vi "PC_COUNT_ALL_SS_1.vi"(0 "Refnum in":T1, 1 "data in":string[][](array[string]), 3 "Array 3":string[](array[string]), 5 "To Date":string, 9 "From Date":string, 11 "error in (no error)":errorcluster, 12 "Station":string[](array[string])=["1", "2", "3", "4", "5", "6"], 14 "Shift":string[](array[string])=["1", "2", "3", "4", "5", "6"]) -> (4 "Refnum out":T1, 6 "data out":string[][](array[string]), 8 "DATE":string[](array[string]), 10 "COUNT":string[](array[string]), 15 "error out":errorcluster)   [LabVIEW 2017]
uses:
  <vilib>/addons/database/Connection.llb/Conn ObjectReference.ctl
  <vilib>/addons/database/NI_Database_API.lvlib
panel:
  in  "STATION":i32[](array[numeric])
  in  "SHIFT":i32[](array[numeric])
  in  "From Date":timestamp
  in  "To Date":timestamp
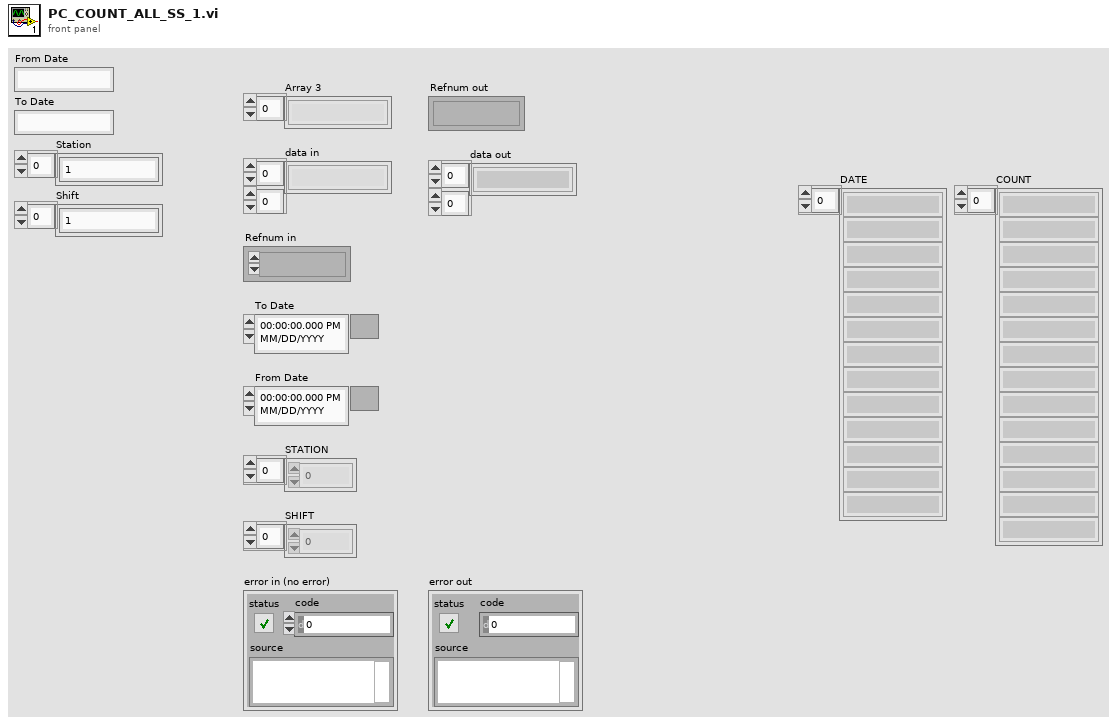
[diagram p1: front panel]
types:
  T1 = typedef "NI_Database_API.lvlib/Conn ObjectReference.ctl" = refnum<k1>
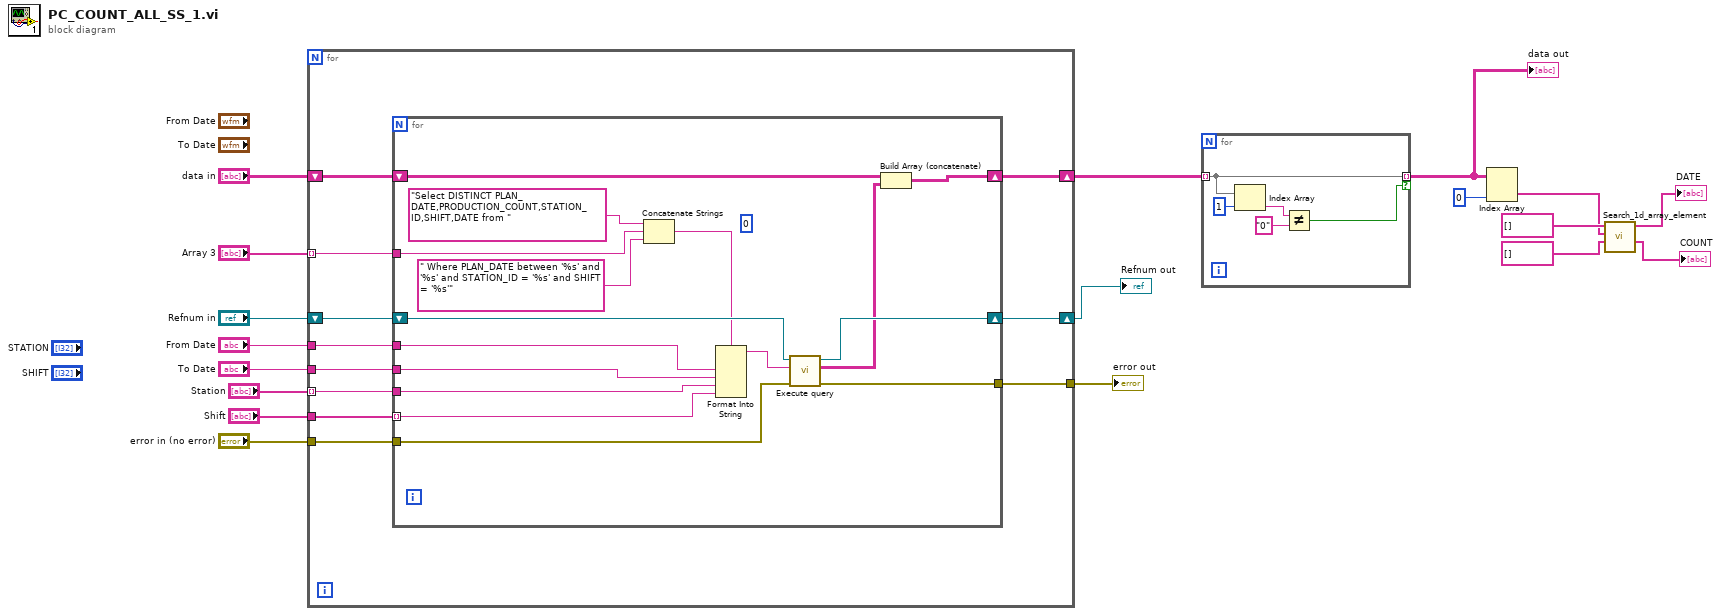
[diagram p0: block diagram]
diagram:
  n1 = for {
    tunnel: "To Date" -> [w29]
    tunnel: "From Date" -> [w28]
    shift-right: [w26] -> w2
    shift-left: "Refnum in" -> [w27]
    tunnel: "Array 3" -> [w25] mode=indexing
    shift-right: [w21] -> w4
    shift-left: "data in" -> [w22]
    tunnel: "error in (no error)" -> [w24]
    tunnel: [w23] -> w18
    tunnel: "Station" -> [w19] mode=indexing
    tunnel: "Shift" -> [w20]
    n2 = for {
      tunnel: w29 -> [w30]
      tunnel: w28 -> [w31]
      tunnel: w25 -> [w43]
      shift-right: [w44] -> w26
      shift-left: w27 -> [w45]
      shift-right: [w39] -> w21
      shift-left: w22 -> [w40]
      tunnel: w20 -> [w32] mode=indexing
      tunnel: w19 -> [w33]
      tunnel: w24 -> [w42]
      tunnel: [w41] -> w23
      (unwired) 0 ("disabled index (col)")
      n3 = Concatenate Strings("Select DISTINCT PLAN_DATE,PRODUCTION_COUNT,STATION_ID,SHIFT,DATE from ", w43, " Where PLAN_DATE between '%s' and '%s' and STATION_ID = '%s' and SHIFT = '%s'") -> (w36:string)
      n4 = Format Into String(format string=w36, w31, w30, w33, w32) -> (resulting string=w38:string)  [unwired: 2 in, 1 out]
      n5 = call "Execute query.vi"("error in (no error)"=w42, "String"=w38, "connection reference"=w45) -> ("error out"=w41:errorcluster, "Table"=w34:string[][], "connection reference 2"=w44:T1)  [unwired: 3 in, 3 out]
      n6 = Build Array (concatenate)(w40, w34) -> (w39:string[][])
    }
  }
  "error out" <- w18
  "Refnum out" <- w2
  n7 = for {
    tunnel: w4 -> [w47] mode=indexing
    tunnel: [w47] -> w3 mode=indexing if=w46
    n8 = Index Array(array=w47, index=1) -> (element=w49:string)
    n9 = Not Equal?(x=w49, y="0") -> (x != y?=w46:bool)
  }
  "data out" <- w3
  n10 = Index Array(array=w3, index (col)=0 ("disabled index (col)")) -> (element=w12:string[])  [unwired: 1 in]
  n11 = call "Search_1d_array_element.vi"("Count in"=string[] [] ("Count"), "BD Date"=w12, "Elements Found in"=string[] [] ("Elements Found")) -> ("Count out"=→"COUNT":string[], "Elements Found out"=→"DATE":string[])  [unwired: 4 in, 1 out]
